vi "myRIO_BRig_Host_endExp_filePath__originalLocation.vi"(10 "input_expPrefix":string, 11 "input_fileName":string) -> (1 "output_filePath":string)   [LabVIEW 2014]
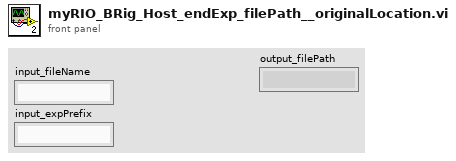
[diagram p1: front panel]
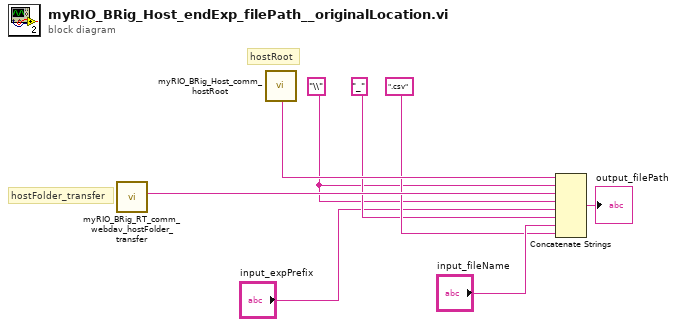
[diagram p0: block diagram]
diagram:
  w3 = "\\" ("string")
  # "hostFolder_transfer"
  # "hostRoot"
  n1 = call "myRIO_BRig_RT_comm_webdav_hostFolder_transfer.vi"() -> ("output_HostFolder"=w8:string)  [unwired: 11 in]
  n2 = call "myRIO_BRig_Host_comm_hostRoot.vi"() -> ("output_hostRoot"=w7:string)  [unwired: 11 in]
  n3 = Concatenate Strings(w7, w3, w8, w3, "input_expPrefix", "_" ("string"), "input_fileName", ".csv" ("string")) -> (→"output_filePath":string)
